vi "HW_Poll_Tracker_2.0.3.vi"(8 "error in":errorcluster, 11 "VISA resource name in":refnum<visa-resource-name>="ASRL3::INSTR") -> (0 "error out":errorcluster, 1 "Read buffer":string, 2 "Parameters output":T1, 3 "VISA resource name out":refnum<visa-resource-name>, 5 "Sensor board size":string)   [LabVIEW 2016]
panel:
  out "Sensors response":string
  out "Port data status":i32
  out "Port data status index":i32
  out "FPS status":i32
  out "Poll records":u32
  out "FPS target index":i32
  out "Matrix mode status":string
  out "Matrix mode index":i32
  out "Coordinate mode status":string
  out "Coordinate mode index":i32
  out "Binary mode status":string
  out "Binary mode index":i32
  out "Array of tokens":string[](array[string])
  out "token index":i32
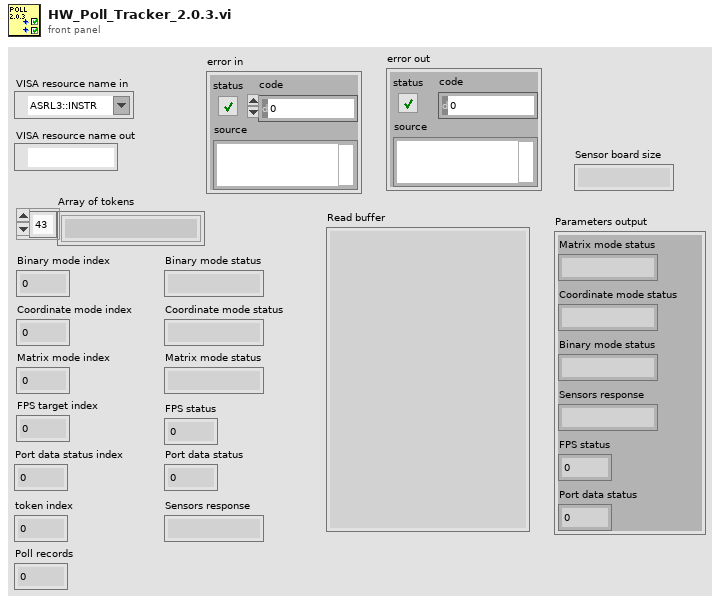
[diagram p1: front panel]
types:
  T1 = cluster{"Matrix mode status":string, "Coordinate mode status":string, "Binary mode status":string, "Sensors response":string, "FPS status":i32, "Port data status":i32}
  T2 = cluster{"token string":string, "token string":string, "token string":string, "trimmed string":string, i32, i32}
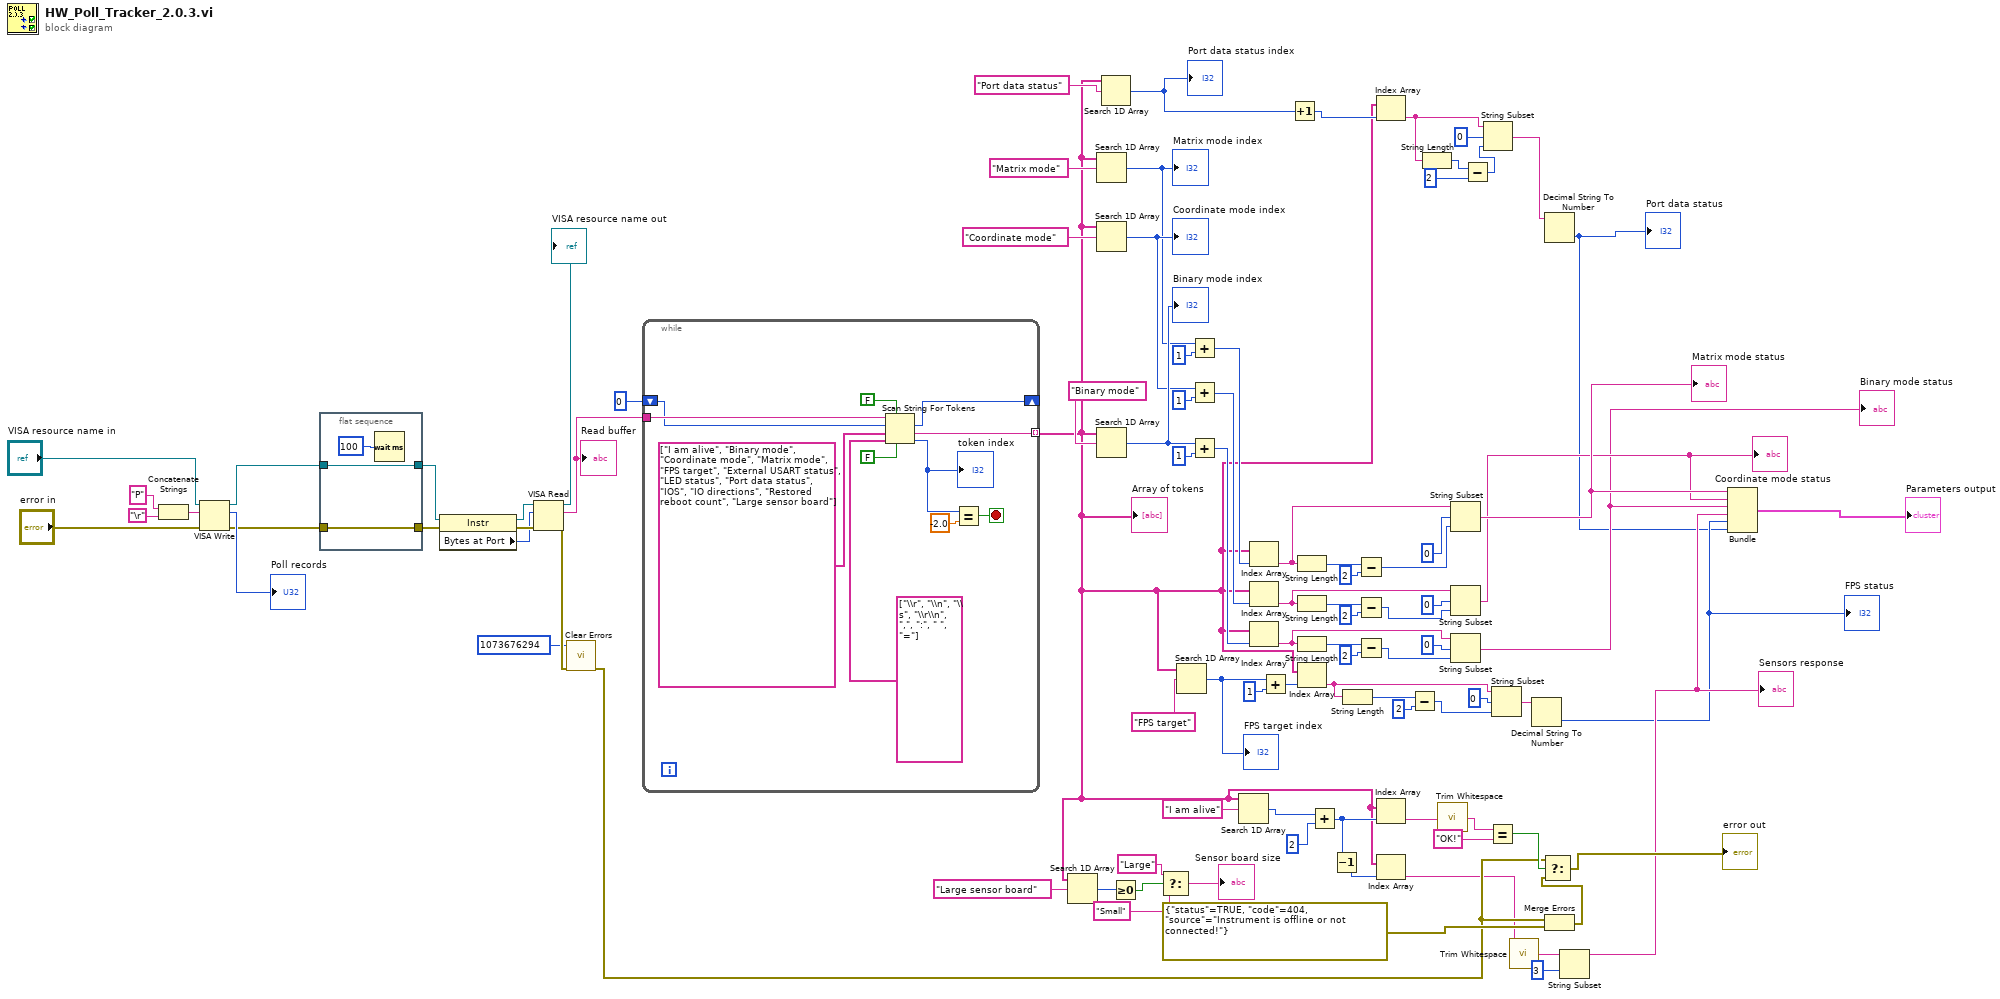
[diagram p0: block diagram]
diagram:
  n1 = Concatenate Strings("P" ("write buffer"), "\r") -> (w92:string)
  n2 = VISA Write(VISA resource name="VISA resource name in", write buffer=w92, error in (no error)="error in") -> (VISA resource name out=w67:refnum<visa-resource-name>, return count=→"Poll records":u32, error out=w65:errorcluster)
  n3 = flat-sequence {
    tunnel: [w96] -> w68
    tunnel: w67 -> [w96]
    tunnel: [w95] -> w66
    tunnel: w65 -> [w95]
    frame #0 {
      n4 = Wait (ms)(milliseconds to wait=u32 100) -> ()  [unwired: 1 out]
    }
  }
  n5 = property class="Instr"(reference=w68, error in=w66) -> (reference out=w90:refnum<visa-resource-name>, error out=w89:errorcluster, "Bytes at Port"=w88:u32)
  n6 = VISA Read(VISA resource name=w90, byte count=w88, error in (no error)=w89) -> (VISA resource name out=→"VISA resource name out":refnum<visa-resource-name>, read buffer=w87:string, error out=w23:errorcluster)  [unwired: 1 out]
  "Read buffer" <- w87
  n7 = call <vilib>:"Clear Errors.vi"("error in (no error)"=w23, "specific error code to clear (0: all)"=1073676294) -> ("error out"=w22:errorcluster)  [unwired: 4 in, 1 out]
  n8 = while {
    tunnel: w87 -> [w108]
    tunnel: [w100] -> w8 mode=indexing
    shift-right: [w99] -> _
    shift-left: 0 ("offset past token") -> [w98]
    stop <- w106 stop-if-true
    n9 = Scan String For Tokens(4:FALSE ("use cached delim/oper data? (F)"), 5:FALSE ("allow empty tokens? (F)"), 6:string[] ["\\r", "\\n", "\\s", "\\r\\n", ",", ":", " ", "="] ("delimiters"), 7:string[] ["I am alive", "Binary mode", "Coordinate mode", "Matrix mode", "FPS target", "External USART status", "LED status", "Port data status", "IOS", "IO directions", "Restored reboot count", "Large sensor board"] ("Tokens"), 8:w98, 9:w108) -> (0:w104:i32, 1:w100:string, 2:w99:i32)  [unwired: 1 out]
    "token index" <- w104
    n10 = Equal?(x=w104, y=-2.0) -> (x = y?=w106:bool)
  }
  "Array of tokens" <- w8
  n11 = Search 1D Array(1D array=w8, element="Large sensor board") -> (index of element=w6:i32)  [unwired: 1 in]
  n12 = Search 1D Array(1D array=w8, element="Matrix mode") -> (index of element=w76:i32)  [unwired: 1 in]
  "Matrix mode index" <- w76
  n13 = Search 1D Array(1D array=w8, element="Coordinate mode") -> (index of element=w80:i32)  [unwired: 1 in]
  "Coordinate mode index" <- w80
  n14 = Search 1D Array(1D array=w8, element="Binary mode") -> (index of element=w84:i32)  [unwired: 1 in]
  "Binary mode index" <- w84
  n15 = Search 1D Array(1D array=w8, element="Port data status") -> (index of element=w41:i32)  [unwired: 1 in]
  "Port data status index" <- w41
  n16 = Greater Or Equal To 0?(x=w6) -> (x >= 0?=w5:bool)
  n17 = Select(t="Large", s=w5, f="Small") -> (s? t:f=→"Sensor board size":string)
  n18 = Search 1D Array(1D array=w8, element="FPS target") -> (index of element=w72:i32)  [unwired: 1 in]
  "FPS target index" <- w72
  n19 = Add(x=w76, y=1) -> (x+y=w77:i32)
  n20 = Add(x=w80, y=1) -> (x+y=w81:i32)
  n21 = Add(x=w84, y=1) -> (x+y=w85:i32)
  n22 = Search 1D Array(1D array=w8, element="I am alive") -> (index of element=w32:i32)  [unwired: 1 in]
  n23 = Index Array(array=w8, index=w77) -> (element=w45:string)
  n24 = Index Array(array=w8, index=w81) -> (element=w43:string)
  n25 = Index Array(array=w8, index=w85) -> (element=w62:string)
  n26 = Add(x=w72, y=1) -> (x+y=w73:i32)
  n27 = Increment(x=w41) -> (x+1=w40:i32)
  n28 = String Length(string=w45) -> (length=w57:i32)
  n29 = String Length(string=w43) -> (length=w48:i32)
  n30 = String Length(string=w62) -> (length=w61:i32)
  n31 = Index Array(array=w8, index=w73) -> (element=w44:string)
  n32 = Add(x=w32, y=2) -> (x+y=w20:i32)
  n33 = Decrement(x=w20) -> (x-1=w19:i32)
  n34 = String Length(string=w44) -> (length=w53:i32)
  n35 = Subtract(x=w57, y=2) -> (x-y=w55:i32)
  n36 = Subtract(x=w48, y=2) -> (x-y=w46:i32)
  n37 = Subtract(x=w61, y=2) -> (x-y=w59:i32)
  n38 = Index Array(array=w8, index=w40) -> (element=w39:string)
  n39 = Index Array(array=w8, index=w20) -> (element=w30:string)
  n40 = Index Array(array=w8, index=w19) -> (element=w18:string)
  n41 = Subtract(x=w53, y=2) -> (x-y=w51:i32)
  n42 = String Length(string=w39) -> (length=w38:i32)
  n43 = call <vilib>:"Trim Whitespace.vi"("string"=w30) -> ("trimmed string"=w29:string)  [unwired: 1 in]
  n44 = String Subset(string=w45, offset (0)=0, length (rest)=w55) -> (substring=w15:string)
  "Matrix mode status" <- w15
  n45 = String Subset(string=w43, offset (0)=0, length (rest)=w46) -> (substring=w14:string)
  "Coordinate mode status" <- w14
  n46 = String Subset(string=w62, offset (0)=0, length (rest)=w59) -> (substring=w13:string)
  "Binary mode status" <- w13
  n47 = Subtract(x=w38, y=2) -> (x-y=w36:i32)
  n48 = String Subset(string=w39, offset (0)=0, length (rest)=w36) -> (substring=w34:string)
  n49 = Equal?(x=w29, y="OK!") -> (x = y?=w27:bool)
  n50 = String Subset(string=w44, offset (0)=0, length (rest)=w51) -> (substring=w50:string)
  n51 = call <vilib>:"Trim Whitespace.vi"("string"=w18) -> ("trimmed string"=w17:string)  [unwired: 1 in]
  n52 = Decimal String To Number(string=w50) -> (number=w11:i32)  [unwired: 2 in, 1 out]
  "FPS status" <- w11
  n53 = Decimal String To Number(string=w34) -> (number=w10:i32)  [unwired: 2 in, 1 out]
  "Port data status" <- w10
  n54 = Merge Errors(w22, errorcluster {"status"=TRUE, "code"=404, "source"="Instrument is offline or not connected!"} ("error in")) -> (w25:errorcluster)
  n55 = Select(t=w22, s=w27, f=w25) -> (s? t:f=→"error out":errorcluster)
  n56 = String Subset(string=w17, offset (0)=3) -> (substring=w12:string)  [unwired: 1 in]
  "Sensors response" <- w12
  n57 = Bundle("token string"=w15, "token string"=w14, "token string"=w13, "trimmed string"=w12, w11, w10) -> (→"Parameters output":T2)  [unwired: 1 in]
